vi "Folder - Get Application Folders Ref.vi"(11 "Pages":refnum<vi>[](array[refnum])) -> (2 "Host Paths":refnum<vi>[](array[refnum]), 3 "Paths":refnum<vi>[](array[refnum]))   [LabVIEW 2013]
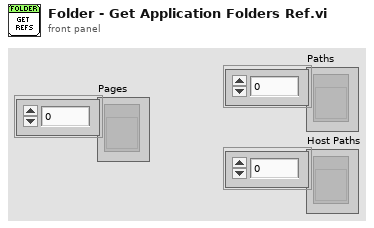
[diagram p1: front panel]
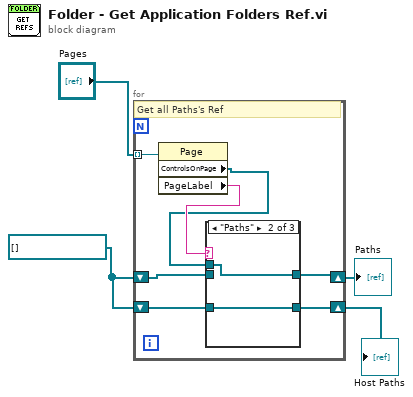
[diagram p0: block diagram]
diagram:
  w3 = refnum<vi>[] [] ("ControlsOnPage")
  n1 = for {
    tunnel: "Pages" -> [w11] mode=indexing
    shift-right: [w5] -> w2
    shift-left: w3 -> [w8]
    shift-right: [w7] -> w1
    shift-left: w3 -> [w6]
    # "Get all Paths's Ref"
    n2 = property class="Page"(reference=w11) -> ("ControlsOnPage"=w9:refnum<vi>[], "PageLabel"=w10:string)  [unwired: 1 in, 2 out]
    n3 = case shown="\"Paths\"" w10 {
      tunnel: w9 -> [_ w15 w17]
      tunnel: w8 -> [w12 _ w16]
      tunnel: [w13 w14 w17] -> w7
      tunnel: w6 -> [w13 w14 _]
      tunnel: [w12 w15 w16] -> w5
      frame "False", Default {
      }
      frame "Paths" {
      }
      frame "Host Paths" {
      }
    }
  }
  "Paths" <- w2
  "Host Paths" <- w1
